vi "Print Console.vi"() -> ()   [LabVIEW 2010]
doc: "이 인쇄 큐 콘솔은 인쇄 작업 제출의 컨트롤을 시뮬레이션하고 처리 중인 인쇄 작업의 상태를 모니터합니다."
uses:
  Print Indicators.ctl
  Print Processing States.ctl
  <vilib>/Utility/error.llb/DialogType.ctl
panel:
  out "인쇄 인디케이터":T1={"대기 중"=TRUE, "초기화 중"=FALSE, "인쇄 중"=FALSE, "작업 수"=0}
  out "큐 인쇄 작업":i32(slide) scale=0.0..25.0
  in  "큐 이벤트":bool
  in  "정지":bool
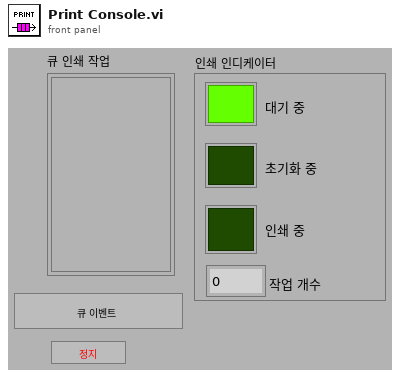
[diagram p1: front panel]
types:
  T1 = typedef "Print Indicators.ctl" = cluster{"대기 중":bool, "초기화 중":bool, "인쇄 중":bool, "작업 수":i32}
  T2 = typedef "DialogType.ctl" = u16
  T3 = typedef "Print Processing States.ctl" = enum16{"대기", "셋업 초기화", "셋업", "인쇄 초기화", "인쇄", "종료"}
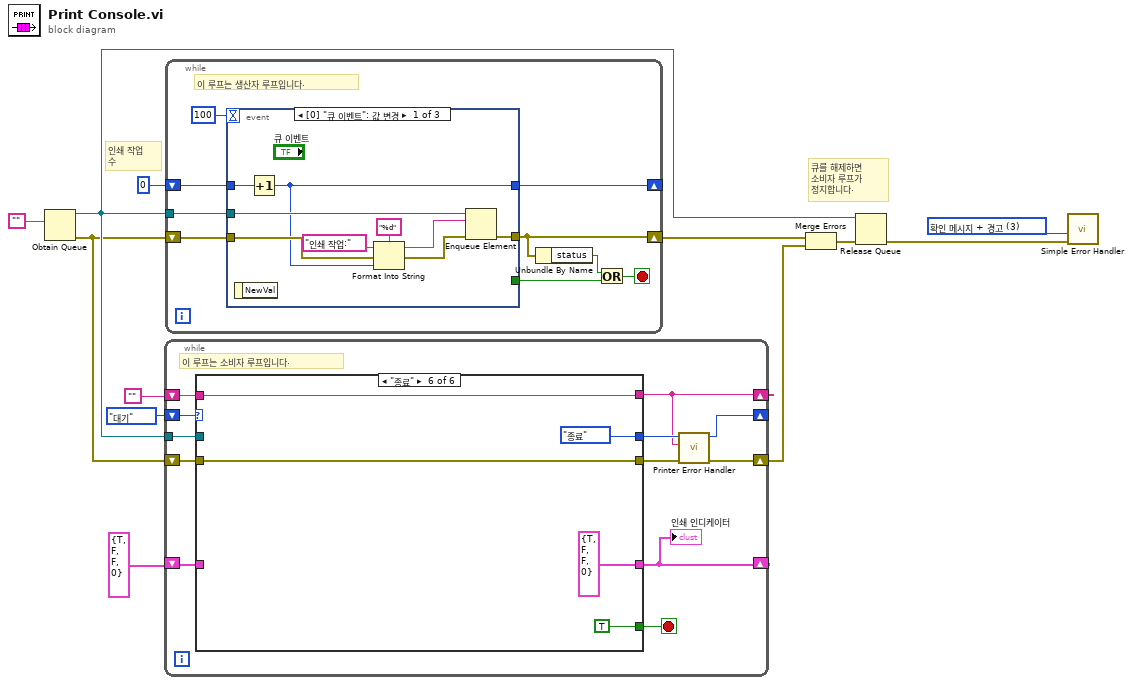
[diagram p0: block diagram]
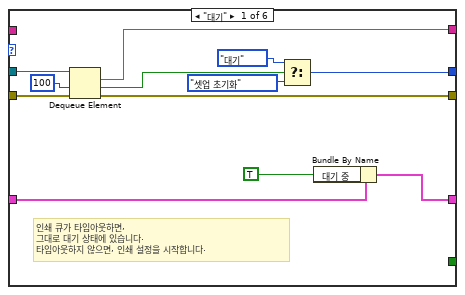
[diagram p2: hidden frame]
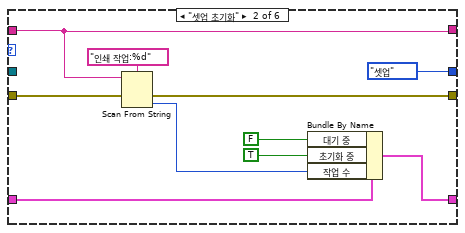
[diagram p3: hidden frame]
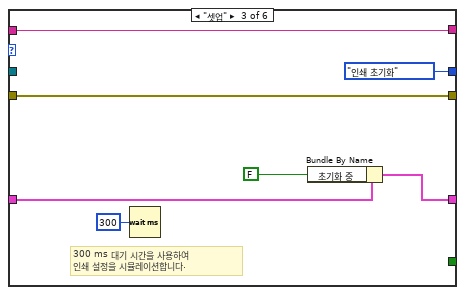
[diagram p4: hidden frame]
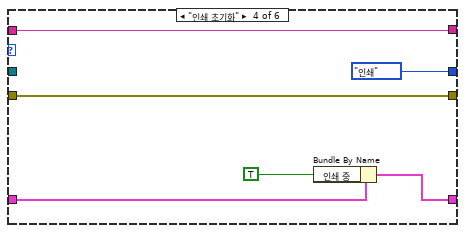
[diagram p5: hidden frame]
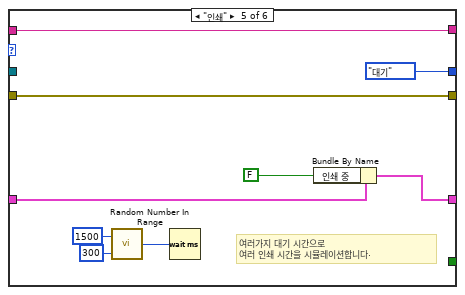
[diagram p6: hidden frame]
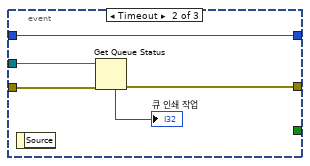
[diagram p7: hidden frame]
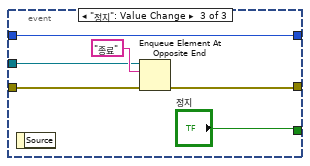
[diagram p8: hidden frame]
diagram:
  w1 = T2 3 items=["대화 상자 없음", "확인 메시지", "메시지 지속 또는 정지", "확인 메시지 + 경고", "지속/정지 + 경고"] ("type of dialog (OK msg:1)")
  # "인쇄 작업\n수"
  # "큐를 해제하면\n소비자 루프가\n정지합니다."
  n1 = Obtain Queue(element data type="") -> (queue out=w11:refnum<queue>, error out=w8:errorcluster)  [unwired: 4 in, 1 out]
  n2 = while {
    tunnel: w11 -> [w24]
    shift-right: [w16] -> _
    shift-left: Print_Processing_States."대기" ("Enum") -> [w23]
    shift-right: [w21] -> _
    shift-left: T1 {"대기 중"=TRUE, "초기화 중"=FALSE, "인쇄 중"=FALSE, "작업 수"=0} ("Print LEDs") -> [w22]
    shift-right: [w18] -> w7
    shift-left: w8 -> [w20]
    shift-right: [w13] -> _
    shift-left: "" -> [w14]
    stop <- w15 stop-if-true
    # "이 루프는 소비자 루프입니다."
    n3 = case shown="\"종료\"" w23 {
      tunnel: w24 -> [w36 _ _ _ _ _]
      tunnel: [w35 w39 w48 w55 w61 w72] -> w19
      tunnel: w22 -> [w30 w45 w52 w58 w67 _]
      tunnel: [w29 w44 w51 w57 w66 T1 {"대기 중"=TRUE, "초기화 중"=FALSE, "인쇄 중"=FALSE, "작업 수"=0} ("Print LEDs")] -> w21
      tunnel: [w27 Print_Processing_States."셋업" ("Enum") Print_Processing_States."인쇄 초기화" ("Enum") Print_Processing_States."인쇄" ("Enum") Print_Processing_States."대기" ("Enum") Print_Processing_States."종료" ("Enum")] -> w17
      tunnel: w20 -> [w26 w41 w48 w55 w61 w72]
      tunnel: [_ _ _ _ _ TRUE] -> w15
      tunnel: [w25 w40 w47 w54 w60 w69] -> w13
      tunnel: w14 -> [_ w40 w47 w54 w60 w69]
      frame "대기" {
        # "인쇄 큐가 타임아웃하면,\n그대로 대기 상태에 있습니다.\n타임아웃하지 않으면, 인쇄 설정을 시작합니다."
        n4 = Dequeue Element(queue=w36, timeout in ms (-1)=100, error in (no error)=w26) -> (element=w25:string, timed out?=w28:bool, error out=w35:errorcluster)  [unwired: 1 out]
        n5 = Select(t=Print_Processing_States."대기" ("Enum"), s=w28, f=Print_Processing_States."셋업 초기화" ("Enum")) -> (s? t:f=w27:T3)
        n6 = Bundle By Name(cluster=w30, "대기 중"=TRUE ("Waiting for\nnew job...")) -> (w29:T1)
      }
      frame "셋업 초기화" {
        n7 = Scan From String(format string="인쇄 작업:%d", input string=w40, error in=w41) -> (error out=w39:errorcluster, output 1=w37:i32)  [unwired: 2 in, 2 out]
        n8 = Bundle By Name(cluster=w45, "대기 중"=FALSE ("Waiting for\nnew job..."), "초기화 중"=TRUE ("Waiting for\nnew job..."), "작업 수"=w37) -> (w44:T1)
      }
      frame "셋업" {
        # "300 ms 대기 시간을 사용하여\n인쇄 설정을 시뮬레이션합니다."
        n9 = Wait (ms)(milliseconds to wait=u32 300) -> ()  [unwired: 1 out]
        n10 = Bundle By Name(cluster=w52, "초기화 중"=FALSE ("Waiting for\nnew job...")) -> (w51:T1)
      }
      frame "인쇄 초기화" {
        n11 = Bundle By Name(cluster=w58, "인쇄 중"=TRUE ("Waiting for\nnew job...")) -> (w57:T1)
      }
      frame "인쇄" {
        # "여러가지 대기 시간으로\n여러 인쇄 시간을 시뮬레이션합니다."
        n12 = call "Random Number In Range.vi"("하위 리미트"=u32 300 ("Lower Limit"), "상위 리미트"=u32 1500 ("Upper Limit")) -> ("임의의 수"=w62:u32)
        n13 = Wait (ms)(milliseconds to wait=w62) -> ()  [unwired: 1 out]
        n14 = Bundle By Name(cluster=w67, "인쇄 중"=FALSE ("Waiting for\nnew job...")) -> (w66:T1)
      }
      frame "종료" {
      }
    }
    "인쇄 인디케이터" <- w21
    n15 = call "Printer Error Handler.vi"("에러 입력(에러 없음)"=w19, "큐 데이터"=w13, "상태"=w17) -> ("에러 출력"=w18:errorcluster, "다음 상태"=w16:T3)  [unwired: 7 in]
  }
  n16 = while {
    shift-right: [w78] -> w6
    shift-left: w8 -> [w81]
    tunnel: w11 -> [w82]
    shift-right: [w74] -> _
    shift-left: 0 -> [w75]
    stop <- w79 stop-if-true
    # "이 루프는 생산자 루프입니다."
    n17 = event shown="[0] \"큐 이벤트\": 값 변경" {
      selector: _ -> [_ _ _]
      dyn-events: _ -> [_ _ _]
      timeout: 100 -> [_ _ _]
      tunnel: w82 -> [w91 w94 w98]
      tunnel: w81 -> [w89 w95 w100]
      tunnel: [w90 w93 w99] -> w78
      tunnel: [_ _ "정지"] -> w80
      tunnel: w75 -> [w85 w92 w97]
      tunnel: [w83 w92 w97] -> w74
      event "큐 이벤트": Value Change {
        n18 = event-data() -> ()  [unwired: 1 in, 1 out]
        n19 = Increment(x=w85) -> (x+1=w83:i32)
        n20 = Format Into String(format string="%d", initial string="인쇄 작업:", error in=w89, w83) -> (resulting string=w84:string, error out=w88:errorcluster)
        n21 = Enqueue Element(queue=w91, element=w84, error in (no error)=w88) -> (error out=w90:errorcluster)  [unwired: 1 in, 2 out]
      }
      event Timeout {
        n22 = event-data() -> ()  [unwired: 1 in, 1 out]
        n23 = Get Queue Status(queue=w94, error in (no error)=w95) -> (error out=w93:errorcluster, # elements in queue=→"큐 인쇄 작업":i32)  [unwired: 1 in, 6 out]
      }
      event "정지": Value Change {
        n24 = event-data() -> ()  [unwired: 1 in, 1 out]
        n25 = Enqueue Element At Opposite End(queue=w98, element="종료", error in (no error)=w100) -> (error out=w99:errorcluster)  [unwired: 1 in, 2 out]
      }
    }
    n26 = Unbundle By Name(w78) -> ("status"=w77:bool)
    n27 = Or(x=w77, y=w80) -> (x .or. y?=w79:bool)
  }
  n28 = Merge Errors(w6, w7) -> (w5:errorcluster)
  n29 = Release Queue(queue=w11, error in (no error)=w5) -> (error out=w4:errorcluster)  [unwired: 1 in, 2 out]
  n30 = call <vilib>:"Simple Error Handler.vi"("type of dialog (OK msg:1)"=w1, "error in (no error)"=w4) -> ()  [unwired: 3 in, 5 out]
